vi "servers.vi"(8 "error in (no error)":errorcluster) -> (0 "error out":errorcluster)   [LabVIEW 2018]
uses:
  Server/Server.lvclass
  RxTx/RxTx.lvclass
  Server/Server.lvclass/Server.ctl
  <vilib>/addons/_JKI Toolkits/Caraya/classes/Assert/Assert Equal Value_Variant.vi
  <vilib>/addons/_JKI Toolkits/Caraya/classes/Assert/Assert Not Error.vi
  <vilib>/addons/_JKI Toolkits/Caraya/classes/Test/Test.lvclass
  <vilib>/addons/_JKI Toolkits/Caraya/classes/Assert/Assert.lvclass
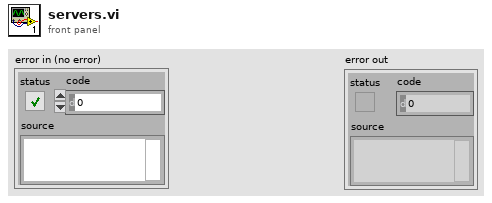
[diagram p1: front panel]
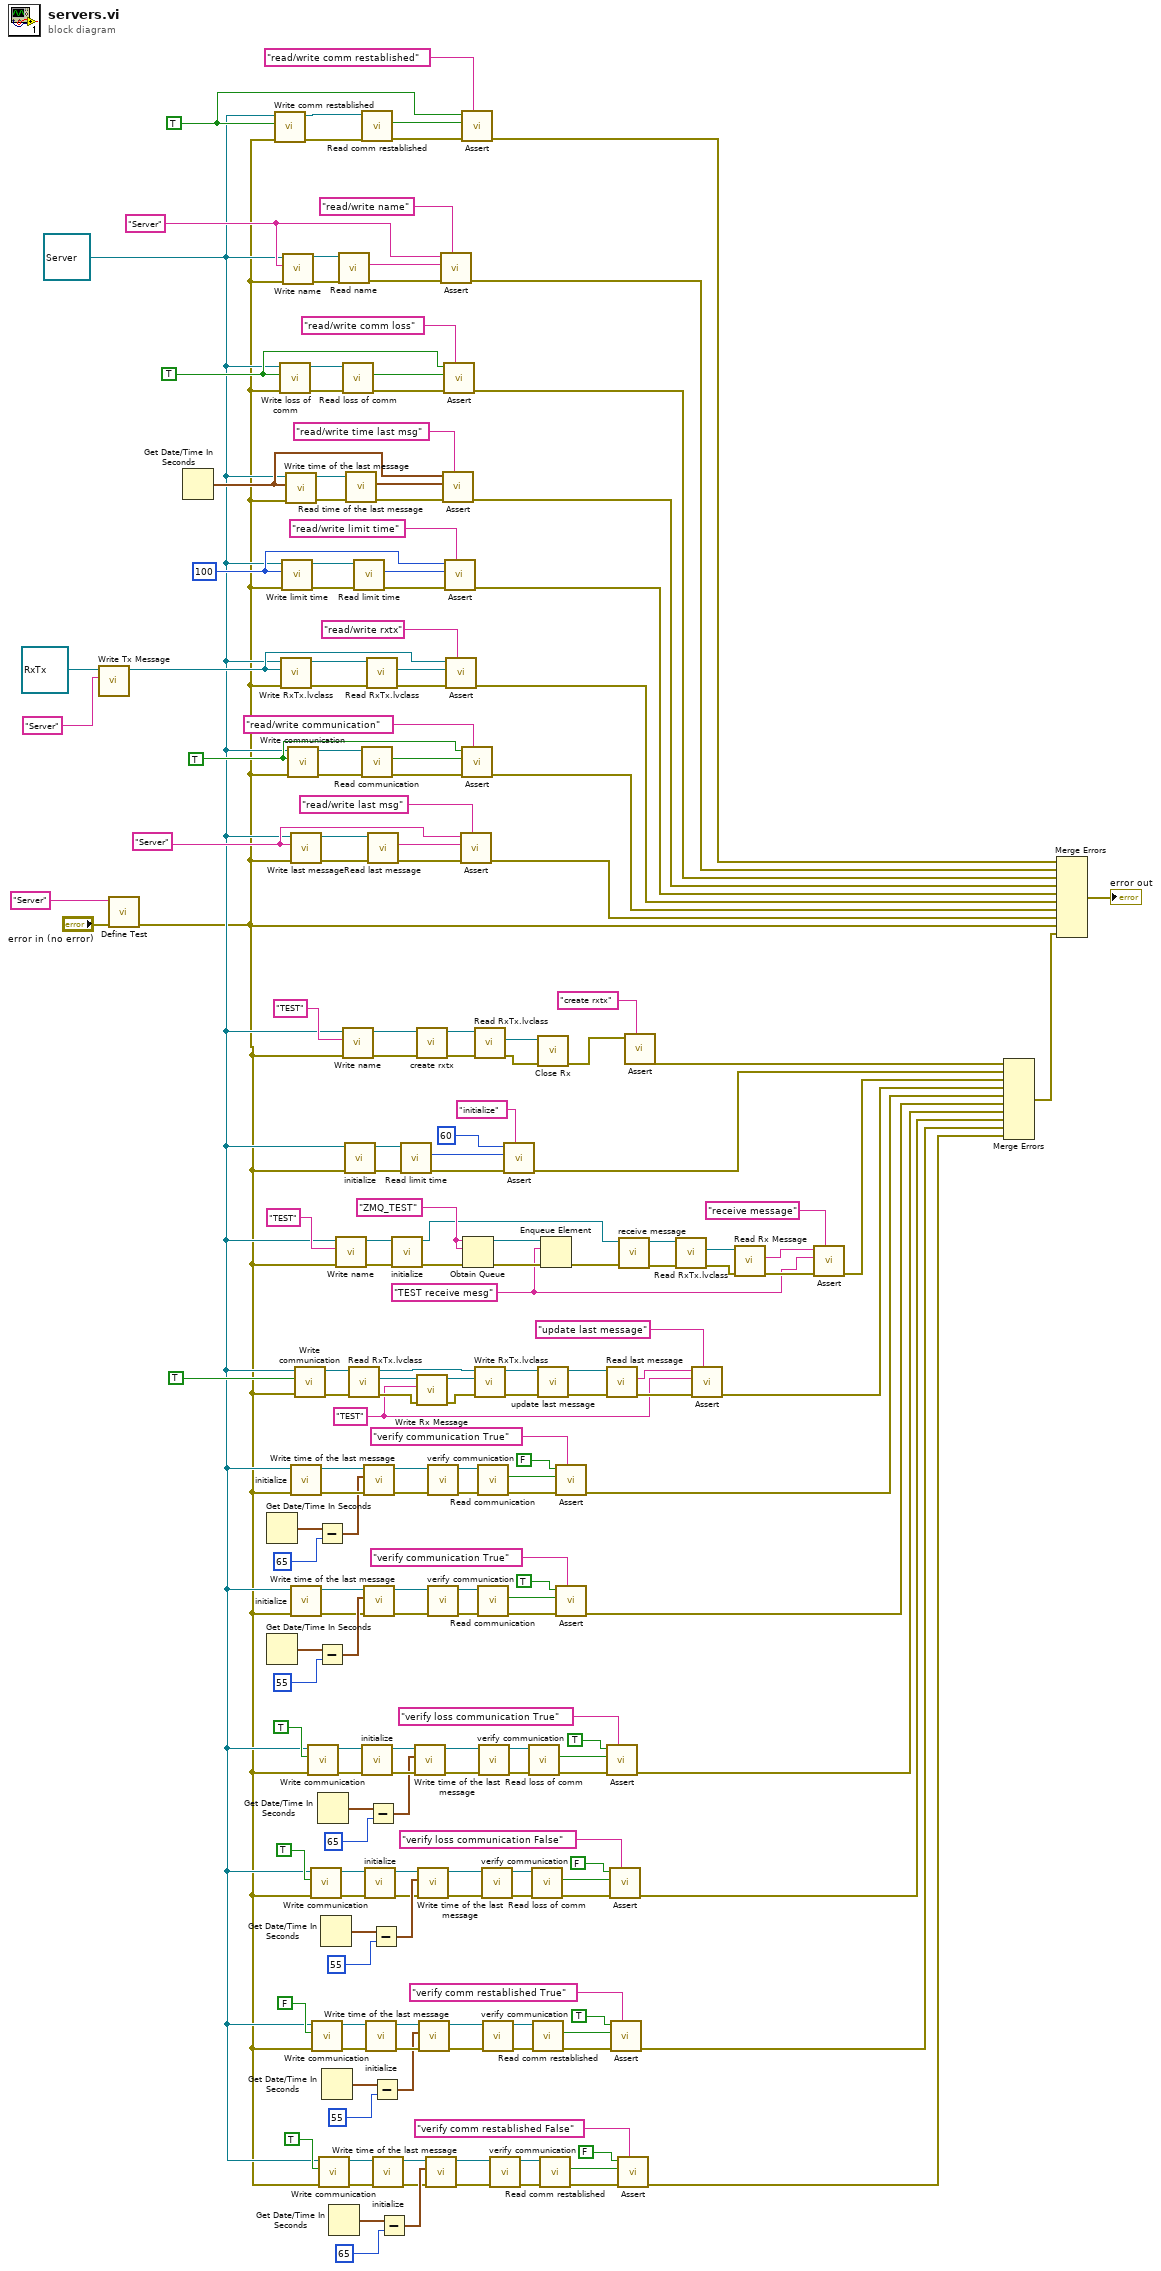
[diagram p0: block diagram]
diagram:
  w100 = "TEST" ("name")
  w118 = "TEST receive mesg" ("name")
  w128 = "ZMQ_TEST" ("name")
  w135 = TRUE ("loss of comm")
  w160 = "Server" ("Label (VI Title)")
  w167 = TRUE ("loss of comm")
  w183 = u16 100 ("limit time")
  w196 = TRUE ("loss of comm")
  w202 = "Server" ("Label (VI Title)")
  w3 = refnum<class "Server.lvclass"> refnum ("Server.lvclass")
  n1 = call "Write Tx Message.vi"("Tx Message"="Server" ("Label (VI Title)"), "RxTx in"=refnum<class "RxTx.lvclass"> refnum ("RxTx.lvclass")) -> ("RxTx out"=w175:refnum<class "RxTx.lvclass">)  [unwired: 8 in, 1 out]
  n2 = call <vilib>:"Define Test.vi"("error in (no error)"="error in (no error)", "Label (VI Title)"="Server") -> ("error out"=w2:errorcluster)  [unwired: 8 in, 1 out]
  n3 = Get Date/Time In Seconds() -> (seconds since 1Jan1904=w191:timestamp)
  n4 = Get Date/Time In Seconds() -> (seconds since 1Jan1904=w96:timestamp)
  n5 = Get Date/Time In Seconds() -> (seconds since 1Jan1904=w74:timestamp)
  n6 = call-dynamic "Write comm restablished.vi"("error in (no error)"=w2, "comm restablished"=w135, "Server in"=w3) -> ("error out"=w140:errorcluster, "Server out"=w139:refnum<class "Server.lvclass">)  [unwired: 7 in]
  n7 = call-dynamic "Write loss of comm.vi"("error in (no error)"=w2, "loss of comm"=w196, "Server in"=w3) -> ("error out"=w207:errorcluster, "Server out"=w206:refnum<class "Server.lvclass">)  [unwired: 7 in]
  n8 = call-dynamic "Write RxTx.lvclass.vi"("error in (no error)"=w2, "RxTx.lvclass"=w175, "Server in"=w3) -> ("error out"=w180:errorcluster, "Server out"=w177:refnum<class "Server.lvclass">)  [unwired: 7 in]
  n9 = call "Write limit time.vi"("error in (no error)"=w2, "limit time"=w183, "Server in"=w3) -> ("error out"=w188:errorcluster, "Server out"=w187:refnum<class "Server.lvclass">)  [unwired: 7 in]
  n10 = call-dynamic "Write name.vi"("error in (no error)"=w2, "name"=w202, "Server in"=w3) -> ("error out"=w209:errorcluster, "Server out"=w208:refnum<class "Server.lvclass">)  [unwired: 7 in]
  n11 = call "Write time of the last message.vi"("error in (no error)"=w2, "time of the last message"=w191, "Server in"=w3) -> ("error out"=w205:errorcluster, "Server out"=w204:refnum<class "Server.lvclass">)  [unwired: 7 in]
  n12 = call-dynamic "Write communication.vi"("error in (no error)"=w2, "communication"=w167, "Server in"=w3) -> ("error out"=w171:errorcluster, "Server out"=w172:refnum<class "Server.lvclass">)  [unwired: 7 in]
  n13 = call-dynamic "Write last message.vi"("error in (no error)"=w2, "last message"=w160, "Server in"=w3) -> ("error out"=w164:errorcluster, "Server out"=w165:refnum<class "Server.lvclass">)  [unwired: 7 in]
  n14 = call "initialize.vi"("error in (no error)"=w2, "Server in"=w3) -> ("error out"=w97:errorcluster, "Server out"=w98:refnum<class "Server.lvclass">)  [unwired: 8 in]
  n15 = call "initialize.vi"("error in (no error)"=w2, "Server in"=w3) -> ("error out"=w73:errorcluster, "Server out"=w72:refnum<class "Server.lvclass">)  [unwired: 8 in]
  n16 = call-dynamic "Write communication.vi"("error in (no error)"=w2, "communication"=TRUE, "Server in"=w3) -> ("error out"=w113:errorcluster, "Server out"=w114:refnum<class "Server.lvclass">)  [unwired: 7 in]
  n17 = call-dynamic "Write communication.vi"("error in (no error)"=w2, "communication"=TRUE, "Server in"=w3) -> ("error out"=w55:errorcluster, "Server out"=w56:refnum<class "Server.lvclass">)  [unwired: 7 in]
  n18 = call-dynamic "Write communication.vi"("error in (no error)"=w2, "communication"=TRUE, "Server in"=w3) -> ("error out"=w52:errorcluster, "Server out"=w51:refnum<class "Server.lvclass">)  [unwired: 7 in]
  n19 = call-dynamic "Write communication.vi"("error in (no error)"=w2, "communication"=FALSE, "Server in"=w3) -> ("error out"=w22:errorcluster, "Server out"=w23:refnum<class "Server.lvclass">)  [unwired: 7 in]
  n20 = Subtract(x=w96, y=65) -> (x-y=w94:timestamp)
  n21 = Subtract(x=w74, y=55) -> (x-y=w76:timestamp)
  n22 = Get Date/Time In Seconds() -> (seconds since 1Jan1904=w68:timestamp)
  n23 = call-dynamic "Write communication.vi"("error in (no error)"=w2, "communication"=TRUE, "Server in"=w3) -> ("error out"=w18:errorcluster, "Server out"=w17:refnum<class "Server.lvclass">)  [unwired: 7 in]
  n24 = Get Date/Time In Seconds() -> (seconds since 1Jan1904=w40:timestamp)
  n25 = Get Date/Time In Seconds() -> (seconds since 1Jan1904=w34:timestamp)
  n26 = Get Date/Time In Seconds() -> (seconds since 1Jan1904=w6:timestamp)
  n27 = call-dynamic "Write name.vi"("error in (no error)"=w2, "name"="TEST", "Server in"=w3) -> ("error out"=w132:errorcluster, "Server out"=w131:refnum<class "Server.lvclass">)  [unwired: 7 in]
  n28 = call-dynamic "Read name.vi"("error in (no error)"=w209, "Server in"=w208) -> ("error out"=w200:errorcluster, "name"=w203:string)  [unwired: 7 in, 1 out]
  n29 = call-dynamic "Read loss of comm.vi"("error in (no error)"=w207, "Server in"=w206) -> ("error out"=w198:errorcluster, "loss of comm"=w197:bool)  [unwired: 7 in, 1 out]
  n30 = call-dynamic "Write name.vi"("error in (no error)"=w2, "name"="TEST", "Server in"=w3) -> ("error out"=w158:errorcluster, "Server out"=w157:refnum<class "Server.lvclass">)  [unwired: 7 in]
  n31 = call "initialize.vi"("error in (no error)"=w2, "Server in"=w3) -> ("error out"=w147:errorcluster, "Server out"=w146:refnum<class "Server.lvclass">)  [unwired: 8 in]
  n32 = call "Read time of the last message.vi"("error in (no error)"=w205, "Server in"=w204) -> ("error out"=w193:errorcluster, "time of the last message"=w192:timestamp)  [unwired: 7 in, 1 out]
  n33 = call "Read RxTx.lvclass.vi"("error in (no error)"=w113, "Server in"=w114) -> ("error out"=w109:errorcluster, "RxTx.lvclass"=w112:refnum<class "RxTx.lvclass">, "Server out"=w108:refnum<class "Server.lvclass">)  [unwired: 7 in]
  n34 = call-dynamic "Read limit time.vi"("error in (no error)"=w188, "Server in"=w187) -> ("error out"=w186:errorcluster, "limit time"=w184:u16)  [unwired: 7 in, 1 out]
  n35 = call-dynamic "Read comm restablished.vi"("error in (no error)"=w140, "Server in"=w139) -> ("error out"=w138:errorcluster, "comm restablished"=w136:bool)  [unwired: 7 in, 1 out]
  n36 = call "Read communication.vi"("error in (no error)"=w171, "Server in"=w172) -> ("error out"=w170:errorcluster, "communication"=w168:bool)  [unwired: 7 in, 1 out]
  n37 = call "initialize.vi"("error in (no error)"=w55, "Server in"=w56) -> ("error out"=w69:errorcluster, "Server out"=w70:refnum<class "Server.lvclass">)  [unwired: 8 in]
  n38 = call "Write time of the last message.vi"("error in (no error)"=w97, "time of the last message"=w94, "Server in"=w98) -> ("error out"=w93:errorcluster, "Server out"=w92:refnum<class "Server.lvclass">)  [unwired: 7 in]
  n39 = call "Write time of the last message.vi"("error in (no error)"=w73, "time of the last message"=w76, "Server in"=w72) -> ("error out"=w77:errorcluster, "Server out"=w78:refnum<class "Server.lvclass">)  [unwired: 7 in]
  n40 = call "initialize.vi"("error in (no error)"=w52, "Server in"=w51) -> ("error out"=w39:errorcluster, "Server out"=w38:refnum<class "Server.lvclass">)  [unwired: 8 in]
  n41 = call "initialize.vi"("error in (no error)"=w22, "Server in"=w23) -> ("error out"=w35:errorcluster, "Server out"=w36:refnum<class "Server.lvclass">)  [unwired: 8 in]
  n42 = call "Read RxTx.lvclass.vi"("error in (no error)"=w180, "Server in"=w177) -> ("error out"=w181:errorcluster, "RxTx.lvclass"=w176:refnum<class "RxTx.lvclass">)  [unwired: 7 in, 1 out]
  n43 = call "Read last message.vi"("error in (no error)"=w164, "Server in"=w165) -> ("error out"=w163:errorcluster, "last message"=w161:string)  [unwired: 7 in, 1 out]
  n44 = Subtract(x=w68, y=65) -> (x-y=w66:timestamp)
  n45 = Subtract(x=w40, y=55) -> (x-y=w42:timestamp)
  n46 = Subtract(x=w34, y=55) -> (x-y=w32:timestamp)
  n47 = call "initialize.vi"("error in (no error)"=w18, "Server in"=w17) -> ("error out"=w5:errorcluster, "Server out"=w4:refnum<class "Server.lvclass">)  [unwired: 8 in]
  n48 = Subtract(x=w6, y=65) -> (x-y=w8:timestamp)
  n49 = call "initialize.vi"("error in (no error)"=w132, "Server in"=w131) -> ("error out"=w129:errorcluster, "Server out"=w125:refnum<class "Server.lvclass">)  [unwired: 8 in]
  n50 = call-dynamic "Read limit time.vi"("error in (no error)"=w147, "Server in"=w146) -> ("error out"=w145:errorcluster, "limit time"=w142:u16)  [unwired: 7 in, 1 out]
  n51 = call "Write time of the last message.vi"("error in (no error)"=w69, "time of the last message"=w66, "Server in"=w70) -> ("error out"=w65:errorcluster, "Server out"=w64:refnum<class "Server.lvclass">)  [unwired: 7 in]
  n52 = call "create rxtx.vi"("error in (no error)"=w158, "Server in"=w157) -> ("error out"=w155:errorcluster, "Server out"=w154:refnum<class "Server.lvclass">)  [unwired: 8 in]
  n53 = call "Write Rx Message.vi"("error in (no error)"=w109, "Rx Message"=w100, "RxTx in"=w112) -> ("error out"=w110:errorcluster, "RxTx out"=w111:refnum<class "RxTx.lvclass">)  [unwired: 7 in]
  n54 = call "Write time of the last message.vi"("error in (no error)"=w39, "time of the last message"=w42, "Server in"=w38) -> ("error out"=w43:errorcluster, "Server out"=w44:refnum<class "Server.lvclass">)  [unwired: 7 in]
  n55 = call "Write time of the last message.vi"("error in (no error)"=w35, "time of the last message"=w32, "Server in"=w36) -> ("error out"=w31:errorcluster, "Server out"=w30:refnum<class "Server.lvclass">)  [unwired: 7 in]
  n56 = call "Write time of the last message.vi"("error in (no error)"=w5, "time of the last message"=w8, "Server in"=w4) -> ("error out"=w9:errorcluster, "Server out"=w10:refnum<class "Server.lvclass">)  [unwired: 7 in]
  n57 = call "verify communication.vi"("error in (no error)"=w93, "Server in"=w92) -> ("error out"=w91:errorcluster, "Server out"=w90:refnum<class "Server.lvclass">)  [unwired: 8 in]
  n58 = call "verify communication.vi"("error in (no error)"=w77, "Server in"=w78) -> ("error out"=w79:errorcluster, "Server out"=w80:refnum<class "Server.lvclass">)  [unwired: 8 in]
  n59 = call-poly <vilib>:"Assert.vi"("Label"="read/write name", "error in (no error)"=w200, "Actual"=w203, "Expected"=w202) -> ("error out"=w199:errorcluster)  [unwired: 6 in, 1 out]
  n60 = call-poly <vilib>:"Assert.vi"("Label"="read/write time last msg", "error in (no error)"=w193, "Actual"=w192, "Expected"=w191) -> ("error out"=w194:errorcluster)  [unwired: 6 in, 1 out]
  n61 = call-poly <vilib>:"Assert.vi"("Label"="read/write comm loss", "error in (no error)"=w198, "Actual"=w197, "Expected"=w196) -> ("error out"=w195:errorcluster)  [unwired: 6 in, 1 out]
  n62 = call-poly <vilib>:"Assert.vi"("Label"="read/write limit time", "error in (no error)"=w186, "Actual"=w184, "Expected"=w183) -> ("error out"=w185:errorcluster)  [unwired: 6 in, 1 out]
  n63 = call-poly <vilib>:"Assert.vi"("Label"="read/write rxtx", "error in (no error)"=w181, "Actual"=w176, "Expected"=w175) -> ("error out"=w173:errorcluster)  [unwired: 6 in, 1 out]
  n64 = call-poly <vilib>:"Assert.vi"("Label"="read/write last msg", "error in (no error)"=w163, "Actual"=w161, "Expected"=w160) -> ("error out"=w162:errorcluster)  [unwired: 6 in, 1 out]
  n65 = call-poly <vilib>:"Assert.vi"("Label"="read/write comm restablished", "error in (no error)"=w138, "Actual"=w136, "Expected"=w135) -> ("error out"=w137:errorcluster)  [unwired: 6 in, 1 out]
  n66 = call-poly <vilib>:"Assert.vi"("Label"="read/write communication", "error in (no error)"=w170, "Actual"=w168, "Expected"=w167) -> ("error out"=w169:errorcluster)  [unwired: 6 in, 1 out]
  n67 = Obtain Queue(name (unnamed)=w128, element data type=w128, error in (no error)=w129) -> (queue out=w127:refnum<queue>, error out=w130:errorcluster)  [unwired: 2 in, 1 out]
  n68 = call "Read RxTx.lvclass.vi"("error in (no error)"=w155, "Server in"=w154) -> ("error out"=w152:errorcluster, "RxTx.lvclass"=w153:refnum<class "RxTx.lvclass">)  [unwired: 7 in, 1 out]
  n69 = call-dynamic "Write RxTx.lvclass.vi"("error in (no error)"=w110, "RxTx.lvclass"=w111, "Server in"=w108) -> ("error out"=w107:errorcluster, "Server out"=w106:refnum<class "Server.lvclass">)  [unwired: 7 in]
  n70 = call "Read communication.vi"("error in (no error)"=w91, "Server in"=w90) -> ("error out"=w89:errorcluster, "communication"=w87:bool)  [unwired: 7 in, 1 out]
  n71 = call "Read communication.vi"("error in (no error)"=w79, "Server in"=w80) -> ("error out"=w81:errorcluster, "communication"=w82:bool)  [unwired: 7 in, 1 out]
  n72 = call "verify communication.vi"("error in (no error)"=w65, "Server in"=w64) -> ("error out"=w63:errorcluster, "Server out"=w62:refnum<class "Server.lvclass">)  [unwired: 8 in]
  n73 = call "verify communication.vi"("error in (no error)"=w43, "Server in"=w44) -> ("error out"=w45:errorcluster, "Server out"=w46:refnum<class "Server.lvclass">)  [unwired: 8 in]
  n74 = call "verify communication.vi"("error in (no error)"=w31, "Server in"=w30) -> ("error out"=w29:errorcluster, "Server out"=w28:refnum<class "Server.lvclass">)  [unwired: 8 in]
  n75 = call "verify communication.vi"("error in (no error)"=w9, "Server in"=w10) -> ("error out"=w11:errorcluster, "Server out"=w12:refnum<class "Server.lvclass">)  [unwired: 8 in]
  n76 = call-poly <vilib>:"Assert.vi"("Label"="initialize" ("Label (VI Title)"), "error in (no error)"=w145, "Actual"=w142, "Expected"=60) -> ("error out"=w144:errorcluster)  [unwired: 6 in, 1 out]
  n77 = call-dynamic "Read loss of comm.vi"("error in (no error)"=w63, "Server in"=w62) -> ("error out"=w61:errorcluster, "loss of comm"=w60:bool)  [unwired: 7 in, 1 out]
  n78 = call-dynamic "Read loss of comm.vi"("error in (no error)"=w45, "Server in"=w46) -> ("error out"=w47:errorcluster, "loss of comm"=w48:bool)  [unwired: 7 in, 1 out]
  n79 = call-dynamic "Read comm restablished.vi"("error in (no error)"=w29, "Server in"=w28) -> ("error out"=w27:errorcluster, "comm restablished"=w26:bool)  [unwired: 7 in, 1 out]
  n80 = call "Close Rx.vi"("error in (no error)"=w152, "RxTx in"=w153) -> ("error out"=w149:errorcluster)  [unwired: 8 in, 1 out]
  n81 = call "update last message.vi"("error in (no error)"=w107, "Server in"=w106) -> ("error out"=w104:errorcluster, "Server out"=w105:refnum<class "Server.lvclass">)  [unwired: 8 in]
  n82 = call-dynamic "Read comm restablished.vi"("error in (no error)"=w11, "Server in"=w12) -> ("error out"=w13:errorcluster, "comm restablished"=w14:bool)  [unwired: 7 in, 1 out]
  n83 = Enqueue Element(queue=w127, element=w118, error in (no error)=w130) -> (error out=w126:errorcluster)  [unwired: 1 in, 2 out]
  n84 = call-poly <vilib>:"Assert.vi"("Label"="verify communication True" ("name"), "error in (no error)"=w89, "Actual"=w87, "Expected"=FALSE) -> ("error out"=w88:errorcluster)  [unwired: 6 in, 1 out]
  n85 = call-poly <vilib>:"Assert.vi"("Label"="verify communication True" ("name"), "error in (no error)"=w81, "Actual"=w82, "Expected"=TRUE) -> ("error out"=w71:errorcluster)  [unwired: 6 in, 1 out]
  n86 = call "Read last message.vi"("error in (no error)"=w104, "Server in"=w105) -> ("error out"=w103:errorcluster, "last message"=w101:string)  [unwired: 7 in, 1 out]
  n87 = call-poly <vilib>:"Assert.vi"("Label"="verify loss communication True" ("name"), "error in (no error)"=w61, "Actual"=w60, "Expected"=TRUE) -> ("error out"=w57:errorcluster)  [unwired: 6 in, 1 out]
  n88 = call-poly <vilib>:"Assert.vi"("Label"="verify loss communication False" ("name"), "error in (no error)"=w47, "Actual"=w48, "Expected"=FALSE) -> ("error out"=w37:errorcluster)  [unwired: 6 in, 1 out]
  n89 = call-poly <vilib>:"Assert.vi"("Label"="verify comm restablished True" ("name"), "error in (no error)"=w27, "Actual"=w26, "Expected"=TRUE) -> ("error out"=w20:errorcluster)  [unwired: 6 in, 1 out]
  n90 = call-poly <vilib>:"Assert.vi"("Label"="verify comm restablished False" ("name"), "error in (no error)"=w13, "Actual"=w14, "Expected"=FALSE) -> ("error out"=w1:errorcluster)  [unwired: 6 in, 1 out]
  n91 = call "receive message.vi"("error in (no error)"=w126, "Server in"=w125) -> ("error out"=w124:errorcluster, "Server out"=w123:refnum<class "Server.lvclass">)  [unwired: 8 in]
  n92 = call-poly <vilib>:"Assert.vi"("Label"="create rxtx" ("Label (VI Title)"), "Not Error?"=w149) -> ("error out"=w150:errorcluster)  [unwired: 8 in, 1 out]
  n93 = call "Read RxTx.lvclass.vi"("error in (no error)"=w124, "Server in"=w123) -> ("error out"=w121:errorcluster, "RxTx.lvclass"=w122:refnum<class "RxTx.lvclass">)  [unwired: 7 in, 1 out]
  n94 = call-poly <vilib>:"Assert.vi"("Label"="update last message" ("name"), "error in (no error)"=w103, "Actual"=w100, "Expected"=w101) -> ("error out"=w102:errorcluster)  [unwired: 6 in, 1 out]
  n95 = call "Read Rx Message.vi"("error in (no error)"=w121, "RxTx in"=w122) -> ("error out"=w120:errorcluster, "Rx Message"=w119:string)  [unwired: 7 in, 1 out]
  n96 = call-poly <vilib>:"Assert.vi"("Label"="receive message" ("name"), "error in (no error)"=w120, "Actual"=w118, "Expected"=w119) -> ("error out"=w116:errorcluster)  [unwired: 6 in, 1 out]
  n97 = Merge Errors(w150, w144, w116, w102, w88, w71, w57, w37, w20, w1) -> (w151:errorcluster)
  n98 = Merge Errors(w137, w199, w195, w194, w185, w173, w169, w162, w2, w151) -> (→"error out":errorcluster)
